vi "Pre Launch Init.vi"(11 "Parent Actor in":refnum<class "Parent Actor.lvclass">) -> (0 "error out":errorcluster, 3 "Parent Actor out":refnum<class "Parent Actor.lvclass">)   [LabVIEW 2012, in "Parent Actor.lvclass"]
doc: "(<B>Filename</B>: Actor Framework.lvlib:Actor.lvclass:Pre Launch Init.vi)\n\nDefines behavior that occurs after the Launch Actor method is invoked but before the actor's Actor Core method begins running.\n\nThe Pre Launch Init method is guaranteed to finish before the Launch Actor method returns to its caller and before the actor itself receives any messages. Any references that the Pre Launch Init method obtains are guaranteed to have the same lifetime as the actor itself. Any errors that the Pre Launch Init method returns will abort the launch.\n\nBy default, this method does nothing. A descendant class may override it to define behavior."
uses:
  Parent Actor.lvclass
  Parent Actor.lvclass/Parent Actor.ctl
  <vilib>/ActorFramework/Actor/Actor.lvclass
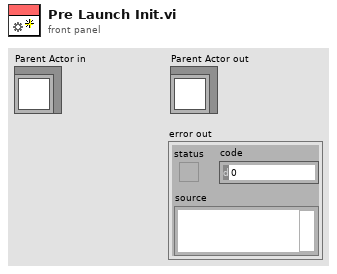
[diagram p1: front panel]
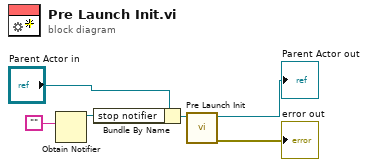
[diagram p0: block diagram]
diagram:
  n1 = Obtain Notifier(notification data type="") -> (notifier out=w2:refnum<notifier>)  [unwired: 3 in, 2 out]
  n2 = Bundle By Name(cluster="Parent Actor in", "stop notifier"=w2) -> (w1:refnum<class "Parent Actor.lvclass">)
  n3 = call-parent "Pre Launch Init.vi"("Actor in"=w1) -> ("error out"=→"error out":errorcluster, "Actor out"=→"Parent Actor out":refnum<class "Parent Actor.lvclass">)  [unwired: 9 in]
